vi "write command into SM.vi"(8 "error in (no error)":errorcluster, 9 "state of the SM":string, 10 "command":string, 11 "Channel in":refnum<class "Channel.lvclass">) -> (0 "error out":errorcluster, 3 "Channel out":refnum<class "Channel.lvclass">)   [LabVIEW 2018, in "Channel.lvclass"]
uses:
  Channel.lvclass
  Channel.lvclass/Channel.ctl
  Log File/Log File.lvclass
  State Machine/State Machine.lvclass
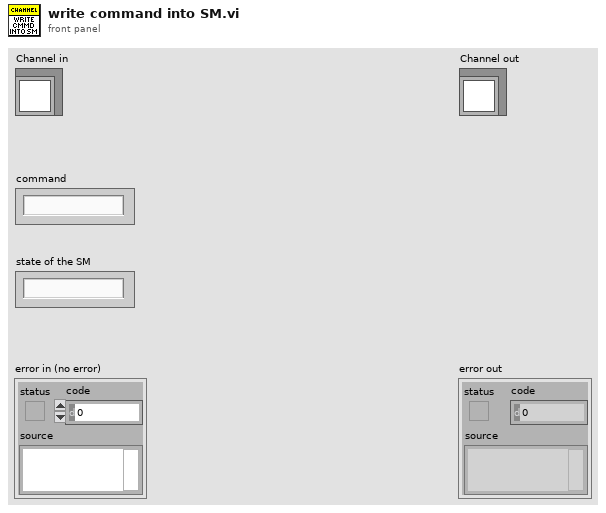
[diagram p1: front panel]
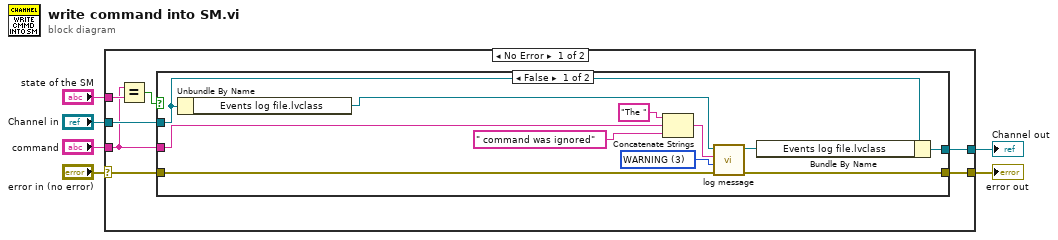
[diagram p0: block diagram]
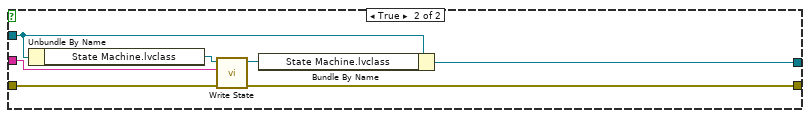
[diagram p2: hidden frame]
diagram:
  n1 = case shown="No Error" "error in (no error)" {
    selector: "error in (no error)" -> [w12 w33]
    tunnel: [w11 w33] -> w5
    tunnel: [w9 w32] -> w3
    tunnel: "Channel in" -> [w10 w32]
    tunnel: "state of the SM" -> [w8 _]
    tunnel: "command" -> [w7 _]
    frame No Error {
      n2 = Equal?(x=w7, y=w8) -> (x = y?=w13:bool)
      n3 = case shown="False" w13 {
        tunnel: w10 -> [w24 w27]
        tunnel: w12 -> [w21 w30]
        tunnel: [w20 w29] -> w11
        tunnel: [w19 w28] -> w9
        tunnel: w7 -> [w17 w25]
        frame False {
          w14 = u16 3 items=[" STATUS ", " DEBBUG ", "  INFO  ", "WARNING ", " ERROR  ", "CRITICAL"] ("log level")
          n4 = Unbundle By Name(w24) -> ("Events log file.lvclass"=w23:refnum<class "Log File.lvclass">)
          n5 = Concatenate Strings("The " ("Message to log"), w17, " command was ignored" ("Message to log")) -> (w15:string)
          n6 = call-dynamic "log message.vi"("error in (no error)"=w21, "log level"=w14, "Message to log"=w15, "Log File in"=w23) -> ("error out"=w20:errorcluster, "Log File out"=w22:refnum<class "Log File.lvclass">)  [unwired: 6 in]
          n7 = Bundle By Name(cluster=w24, "Events log file.lvclass"=w22) -> (w19:refnum<class "Channel.lvclass">)
        }
        frame True {
          n8 = Unbundle By Name(w27) -> ("State Machine.lvclass"=w26:refnum<class "State Machine.lvclass">)
          n9 = call-dynamic "Write State.vi"("error in (no error)"=w30, "State"=w25, "State Machine in"=w26) -> ("error out"=w29:errorcluster, "State Machine out"=w31:refnum<class "State Machine.lvclass">)  [unwired: 7 in]
          n10 = Bundle By Name(cluster=w27, "State Machine.lvclass"=w31) -> (w28:refnum<class "Channel.lvclass">)
        }
      }
    }
    frame Error {
    }
  }
  "error out" <- w5
  "Channel out" <- w3
